vi "DCMotor_GetAndymarkRs775_125.vi"(11 "Num Motors":i32=1) -> (3 "DCMOTOR":T1 {"Jr_KgM2" format="%13.5p"; "L_H" format="%13.5p"; "Kt_NMPerAmp" format="%13.5p"; "KvINV_RadPerSecPerVolt" format="%13.5p"; "R_Ohms" format="%13.5p"; "FreeSpeed_RadPerSec" format="%13.5p"; "FreeCurrent_Amps" format="%13.5p"; "StallCurrent_Amps" format="%13.5p"; "StallTorque_NM" format="%13.5p"; "nominalVoltage_Volts" format="%13.5p"})   [LabVIEW 2019, in "Trajectory_Library.lvlib"]
doc: "Creates a new DC MOTOR data cluster with the specified values. for a set of AndyMark Rs775-125 motors. \n\nInputs: \n - Num Motors -- The number of motors used together in this sytem driving the same load.\n\nOutputs:\n - DCMOTOR -- Cluster containing the motor modeling constants for this set of motors."
uses:
  Trajectory_Library.lvlib
  TypeDef/DCMOTOR.CTL
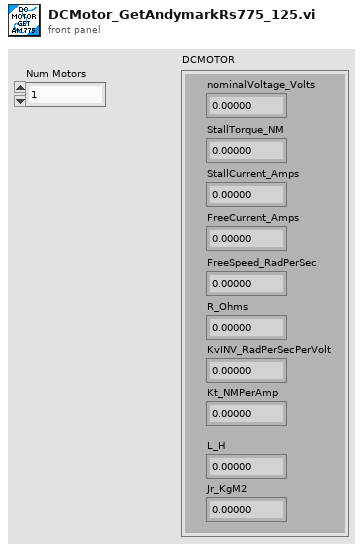
[diagram p1: front panel]
types:
  T1 = typedef "Trajectory_Library.lvlib/DCMOTOR.CTL" = cluster{"nominalVoltage_Volts":dbl, "StallTorque_NM":dbl, "StallCurrent_Amps":dbl, "FreeCurrent_Amps":dbl, "FreeSpeed_RadPerSec":dbl, "R_Ohms":dbl, "KvINV_RadPerSecPerVolt":dbl, "Kt_NMPerAmp":dbl, "L_H":dbl, "Jr_KgM2":dbl}
  T2 = typedef "WPILib_Math.lvlib/DCMOTOR.CTL" = cluster{"nominalVoltage_Volts":dbl, "StallTorque_NM":dbl, "StallCurrent_Amps":dbl, "FreeCurrent_Amps":dbl, "FreeSpeed_RadPerSec":dbl, "R_Ohms":dbl, "KvINV_RadPerSecPerVolt":dbl, "Kt_NMPerAmp":dbl, "L_H":dbl, "Jr_KgM2":dbl}
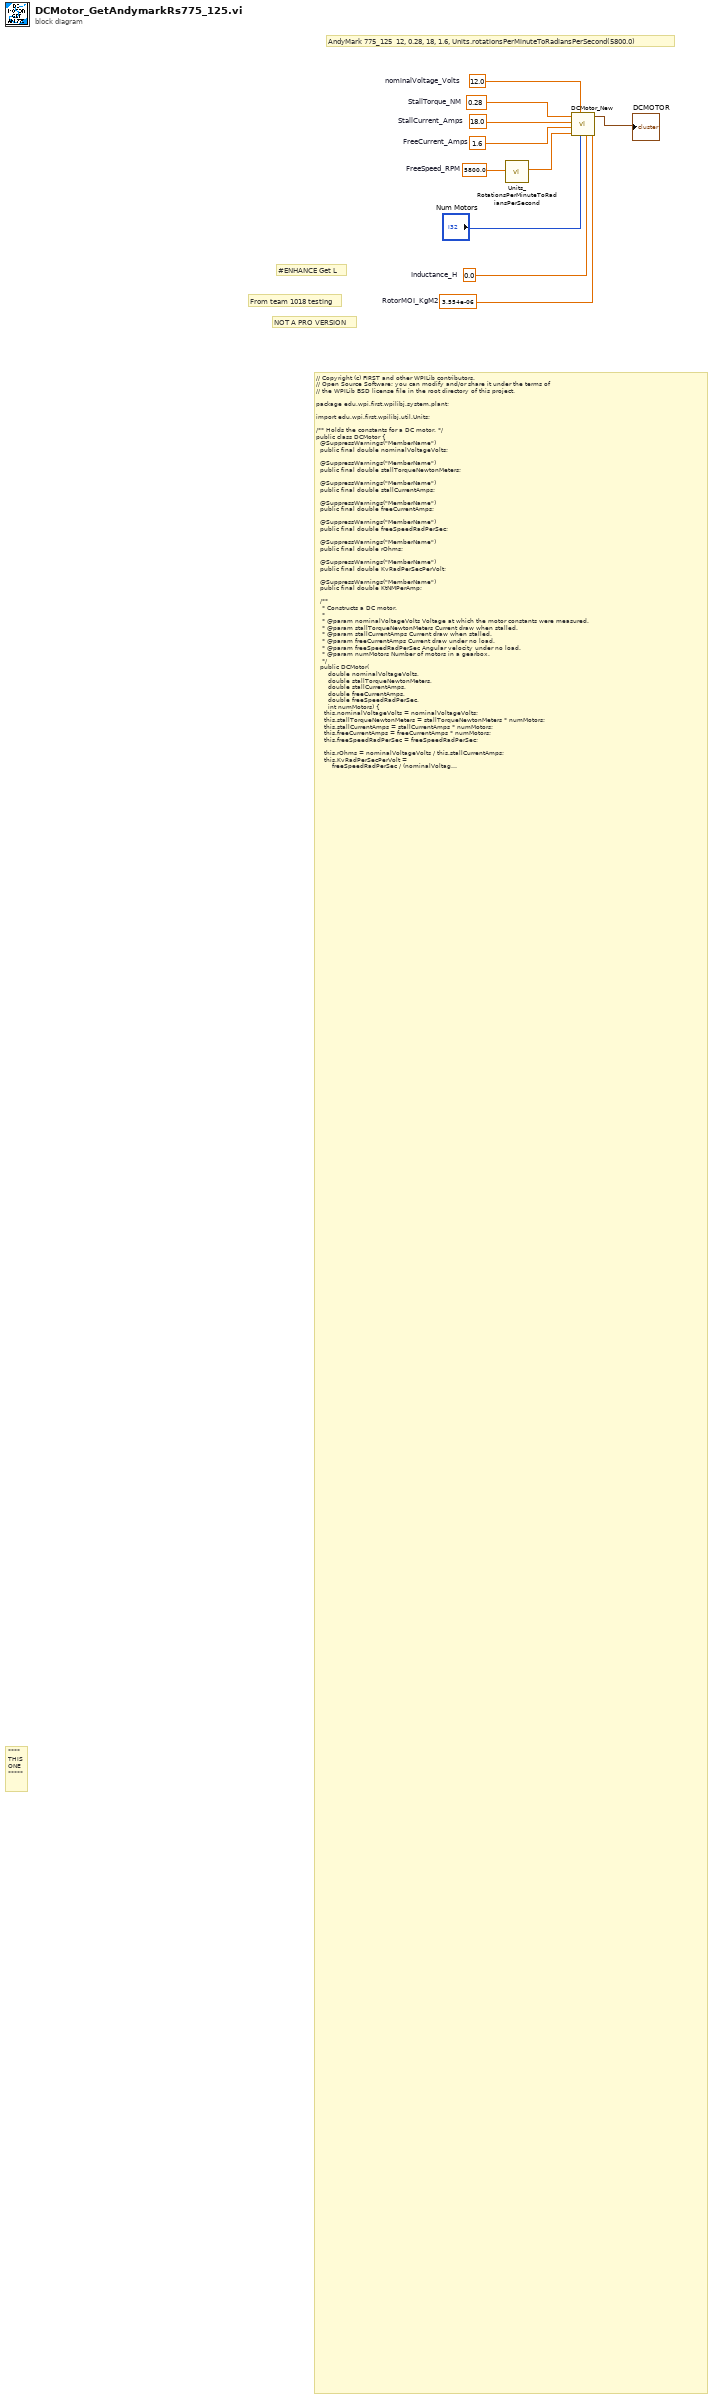
[diagram p0: block diagram]
diagram:
  w1 = 3.554e-06  # RotorMOI_KgM2
  w2 = 0.0  # Inductance_H
  w4 = 5800.0  # FreeSpeed_RPM
  w5 = 1.6  # FreeCurrent_Amps
  w6 = 18.0  # StallCurrent_Amps
  w7 = 0.28  # StallTorque_NM
  w8 = 12.0  # nominalVoltage_Volts
  # "NOT A PRO VERSION"
  # "#ENHANCE Get L"
  # "From team 1018 testing"
  # "AndyMark 775_125  12, 0.28, 18, 1.6, Units.rotationsPerMinuteToRadiansPerSecond(5800.0)"
  # "// Copyright (c) FIRST and other WPILib contributors.\n// Open Source Software; you can modify and/or share it under the terms of\n// the WPILib BSD license file in the root directory of this project.\n\npackage edu.wpi.first.wpilibj.system.plant;\n\nimport edu.wpi.first.wpilibj.util.Units;\n\n/** Holds the constants for a DC motor. */\npublic class DCMotor {\n  @SuppressWarnings(\"MemberName\")\n  public final double nominalVoltageVolts;\n\n  @SuppressWarnings(\"MemberName\")\n  public final double stallTorqueNewtonMeters;\n\n  @SuppressWarnings(\"MemberName\")\n  public final double stallCurrentAmps;\n\n  @SuppressWarnings(\"MemberName\")\n  public final double freeCurrentAmps;\n\n  @SuppressWarnings(\"MemberName\")\n  public final double freeSpeedRadPerSec;\n\n  @SuppressWarnings(\"MemberName\")\n  public final double rOhms;\n\n  @SuppressWarnings(\"MemberName\")\n  public final double KvRadPerSecPerVolt;\n\n  @SuppressWarnings(\"MemberName\")\n  public final double KtNMPerAmp;\n\n  /**\n   * Constructs a DC motor.\n   *\n   * @param nominalVoltageVolts Voltage at which the motor constants were measured.\n   * @param stallTorqueNewtonMeters Current draw when stalled.\n   * @param stallCurrentAmps Current draw when stalled.\n   * @param freeCurrentAmps Current draw under no load.\n   * @param freeSpeedRadPerSec Angular velocity under no load.\n   * @param numMotors Number of motors in a gearbox.\n   */\n  public DCMotor(\n      double nominalVoltageVolts,\n      double stallTorqueNewtonMeters,\n      double stallCurrentAmps,\n      double freeCurrentAmps,\n      double freeSpeedRadPerSec,\n      int numMotors) {\n    this.nominalVoltageVolts = nominalVoltageVolts;\n    this.stallTorqueNewtonMeters = stallTorqueNewtonMeters * numMotors;\n    this.stallCurrentAmps = stallCurrentAmps * numMotors;\n    this.freeCurrentAmps = freeCurrentAmps * numMotors;\n    this.freeSpeedRadPerSec = freeSpeedRadPerSec;\n\n    this.rOhms = nominalVoltageVolts / this.stallCurrentAmps;\n    this.KvRadPerSecPerVolt =\n        freeSpeedRadPerSec / (nominalVoltageVolts - rOhms * this.freeCurrentAmps);\n    this.KtNMPerAmp = this.stallTorqueNewtonMeters / this.stallCurrentAmps;\n  }\n\n  /**\n   * Estimate the current being drawn by this motor.\n   *\n   * @param speedRadiansPerSec The speed of the rotor.\n   * @param voltageInputVolts The input voltage.\n   */\n  public double getCurrent(double speedRadiansPerSec, double voltageInputVolts) {\n    return -1.0 / KvRadPerSecPerVolt / rOhms * speedRadiansPerSec + 1.0 / rOhms * voltageInputVolts;\n  }\n\n  /**\n   * Return a gearbox of CIM motors.\n   *\n   * @param numMotors Number of motors in the gearbox.\n   */\n  public static DCMotor getCIM(int numMotors) {\n    return new DCMotor(\n        12, 2.42, 133, 2.7, Units.rotationsPerMinuteToRadiansPerSecond(5310), numMotors);\n  }\n\n  /**\n   * Return a gearbox of 775Pro motors.\n   *\n   * @param numMotors Number of motors in the gearbox.\n   */\n  public static DCMotor getVex775Pro(int numMotors) {\n    return new DCMotor(\n        12, 0.71, 134, 0.7, Units.rotationsPerMinuteToRadiansPerSecond(18730), numMotors);\n  }\n\n  /**\n   * Return a gearbox of NEO motors.\n   *\n   * @param numMotors Number of motors in the gearbox.\n   */\n  public static DCMotor getNEO(int numMotors) {\n    return new DCMotor(\n        12, 2.6, 105, 1.8, Units.rotationsPerMinuteToRadiansPerSecond(5676), numMotors);\n  }\n\n  /**\n   * Return a gearbox of MiniCIM motors.\n   *\n   * @param numMotors Number of motors in the gearbox.\n   */\n  public static DCMotor getMiniCIM(int numMotors) {\n    return new DCMotor(\n        12, 1.41, 89, 3, Units.rotationsPerMinuteToRadiansPerSecond(5840), numMotors);\n  }\n\n  /**\n   * Return a gearbox of Bag motors.\n   *\n   * @param numMotors Number of motors in the gearbox.\n   */\n  public static DCMotor getBag(int numMotors) {\n    return new DCMotor(\n        12, 0.43, 53, 1.8, Units.rotationsPerMinuteToRadiansPerSecond(13180), numMotors);\n  }\n\n  /**\n   * Return a gearbox of Andymark RS775-125 motors.\n   *\n   * @param numMotors Number of motors in the gearbox.\n   */\n  public static DCMotor getAndymarkRs775_125(int numMotors) {\n    return new DCMotor(\n        12, 0.28, 18, 1.6, Units.rotationsPerMinuteToRadiansPerSecond(5800.0), numMotors);\n  }\n\n  /**\n   * Return a gearbox of Banebots RS775 motors.\n   *\n   * @param numMotors Number of motors in the gearbox.\n   */\n  public static DCMotor getBanebotsRs775(int numMotors) {\n    return new DCMotor(\n        12, 0.72, 97, 2.7, Units.rotationsPerMinuteToRadiansPerSecond(13050.0), numMotors);\n  }\n\n  /**\n   * Return a gearbox of Andymark 9015 motors.\n   *\n   * @param numMotors Number of motors in the gearbox.\n   */\n  public static DCMotor getAndymark9015(int numMotors) {\n    return new DCMotor(\n        12, 0.36, 71, 3.7, Units.rotationsPerMinuteToRadiansPerSecond(14270.0), numMotors);\n  }\n\n  /**\n   * Return a gearbox of Banebots RS 550 motors.\n   *\n   * @param numMotors Number of motors in the gearbox.\n   */\n  public static DCMotor getBanebotsRs550(int numMotors) {\n    return new DCMotor(\n        12, 0.38, 84, 0.4, Units.rotationsPerMinuteToRadiansPerSecond(19000.0), numMotors);\n  }\n\n  /**\n   * Return a gearbox of Neo 550 motors.\n   *\n   * @param numMotors Number of motors in the gearbox.\n   */\n  public static DCMotor getNeo550(int numMotors) {\n    return new DCMotor(\n        12, 0.97, 100, 1.4, Units.rotationsPerMinuteToRadiansPerSecond(11000.0), numMotors);\n  }\n\n  /**\n   * Return a gearbox of Falcon 500 motors.\n   *\n   * @param numMotors Number of motors in the gearbox.\n   */\n  public static DCMotor getFalcon500(int numMotors) {\n    return new DCMotor(\n        12, 4.69, 257, 1.5, Units.rotationsPerMinuteToRadiansPerSecond(6380.0), numMotors);\n  }\n}"
  # "****\nTHIS\nONE\n*****"
  n1 = call "Units_RotationsPerMinuteToRadiansPerSecond.vi"("RotationsPerMinute"=w4) -> ("RadiansPerSecond"=w3:dbl)  [unwired: 10 in]
  n2 = call "DCMotor_New.vi"("RotorMOI_KgM2"=w1, "Inductance_H"=w2, "Num Motors"="Num Motors", "nominalVoltage_Volts"=w8, "FreeSpeed_RadPerSec"=w3, "FreeCurrent_Amps"=w5, "StallCurrent_Amps"=w6, "StallTorque_NM"=w7) -> ("DCMOTOR"=→"DCMOTOR":T2)  [unwired: 3 in]
